vi "Translate triangle.vi"(1 "Translation vector (dx, dy, dz)":sgl[](array[numeric]), 2 "Triangle in":T1) -> (0 "Triangle out":T1)   [LabVIEW 2014]
uses:
  Typedefs/Triangle.ctl
panel:
  # "PN 13/01/2015"
  # "Vertices"
  # "Edges"
  # "Unit normal"
  # "pre-store"
  # "Vertices"
  # "Edges"
  # "Unit normal"
  # "pre-store"
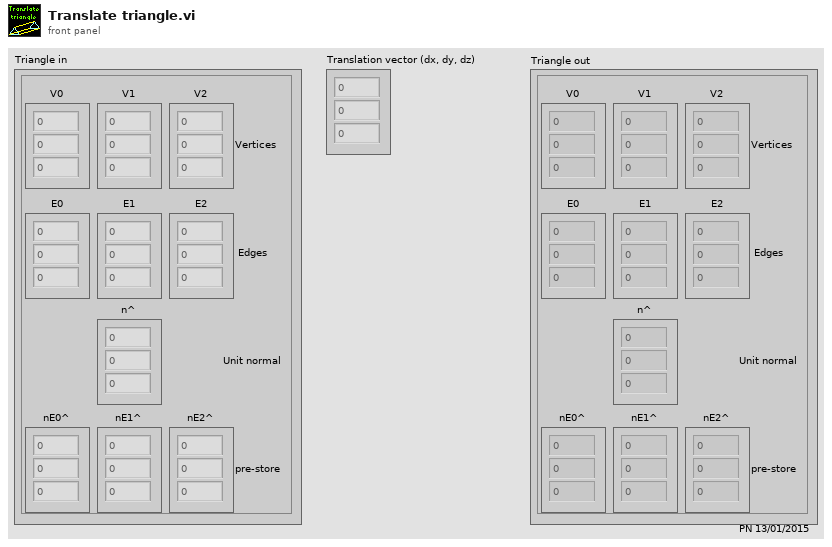
[diagram p1: front panel]
types:
  T1 = typedef "Triangle.ctl" = cluster{"V0":sgl[], "V1":sgl[], "V2":sgl[], "E0":sgl[], "E1":sgl[], "E2":sgl[], "n^":sgl[], "nE0^":sgl[], "nE1^":sgl[], "nE2^":sgl[]}
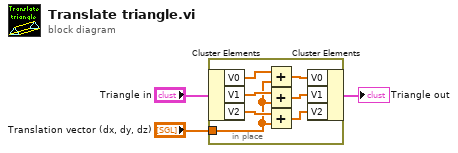
[diagram p0: block diagram]
diagram:
  n1 = in-place {
    in-place-border: "Translation vector (dx, dy, dz)" -> [w6]
    n2 = in-place-cluster #1("Triangle in") -> ("V0"=w10:sgl[], "V1"=w8:sgl[], "V2"=w7:sgl[])
    n3 = Add(x=w10, y=w6) -> (x+y=w9:sgl[])
    n4 = Add(x=w8, y=w6) -> (x+y=w4:sgl[])
    n5 = Add(x=w7, y=w6) -> (x+y=w5:sgl[])
    n6 = in-place-cluster #1("V0"=w9, "V1"=w4, "V2"=w5) -> (→"Triangle out":T1)
  }
